vi "FPGA VI_16 Channels.vi"() -> ()   [LabVIEW 2015]
uses:
  Types/Injector.Timing.ctl
  Types/Injection.Core.Settings.ctl
  Types/Injection.Global.Settings.ctl
  <vilib>/Platform/TimedLoop/XDataNode/timing_clust.ctl
  <vilib>/Platform/TimedLoop/XDataNode/nitl_modes.ctl
  <vilib>/Platform/TimedLoop/XDataNode/wakeup.ctl
  Types/Injection.Core.Internal.Settings.ctl
  <vilib>/rvi/Emulation/niFpgaGetClockAttributes.vi
  <vilib>/rvi/Emulation/niFpgaSctlEmulationGetInTimedLoop.vi
  <vilib>/rvi/Emulation/niFpgaEmulationReportErrorSimple.vi
  <vilib>/rvi/eio/common/nirviEmuTemplateMethod_errors.vi
  <vilib>/rvi/Emulation/niFpgaCriticalErrorInLSC.vi
  <vilib>/rvi/DataTransferAndStorage/Container/Common/niFpgaContainerExecOnDevCompGetState.vi
  <vilib>/rvi/Emulation/niFpgaEmulationIsFPGAContextNoSignature.vi
  <vilib>/rvi/errors/niFpgaSetErrorForExecOnDevCompSimple.vi
  <vilib>/rvi/eio/common/nirviEmuReportErrorAndStop.vi
  <vilib>/rvi/DataTransferAndStorage/Container/Common/niFpgaContainerGetUniqueNameForEmu.vi
  <vilib>/rvi/FIFO/Fifo_Resource/nirvififoEmulationSetSize.vi
  <vilib>/rvi/FIFO/Fifo_Resource/nirviFifoEmulationQueueMgr.vi
  <instcachedir>/0/nirviFifoEmulationQueueMgr_E5CAEC123FF24DC58D834DCA3CDAA9B5.lvgen/nirviFifoEmulationQueueMgr_E5CAEC123FF24DC58D834DCA3CDAA9B5_010.vi
  <vilib>/rvi/FIFO/Fifo_Resource/nirvififoEmulationDetermineInputValidOut.vi
  <vilib>/rvi/FIFO/Fifo_Resource/nirvififoEmulationCreateLock.vi
  <vilib>/rvi/Emulation/niFpgaProcessEmulError.vi
  <vilib>/rvi/FIFO/Fifo_Resource/nirvififoEmulationObtainLock.vi
  <vilib>/rvi/FIFO/Fifo_Resource/nirvififoEmulationReleaseLock.vi
  <vilib>/rvi/occurrence/nirviWaitOnOccurrenceBase.vi
  <vilib>/rvi/errors/nirviReportUnexpectedCaseInternalError.vi
  <vilib>/rvi/errors/nirviReportUnexpectedCaseInternalError (U32).vi
  <vilib>/Utility/error.llb/Clear Errors.vi
  <vilib>/rvi/interface/RandomDataEmulation/niFpgaRandomDataHandleErrors.vi
  <instcachedir>/0/nirviFifoEmulationQueueMgr_E5CAEC123FF24DC58D834DCA3CDAA9B5.lvgen/nirviFifoEmulationQueueMgr_E5CAEC123FF24DC58D834DCA3CDAA9B5_008.vi
  <vilib>/eio/EIONode/EIONode.xnode
  <vilib>/Platform/TimedLoop/XDataNode/XDataNode.xnode
  <vilib>/rvi/DataTransferAndStorage/Container/XNode/niFpgaContainer.xnode
  <vilib>/rvi/FIFO/Fifo_Resource/niFpgaFifoEmulationRefIn.vi
  <vilib>/rvi/interface/RandomDataEmulation/nirviRandomDataFpgaReadWriteTemplate.vi
  <vilib>/Platform/TimedLoop/XDataNode/XDNodeRunTimeDep.lvlib
panel:
  in  "Settings.Index12.Injector12":T1
  in  "Settings.Index13.Injector13":T1
  in  "Settings.Index14.Injector14":T1
  in  "Settings.Index15.Injector15":T1
  in  "Settings.Index6.Injector6":T1
  in  "Settings.Index7.Injector7":T1
  in  "Settings.Index8.Injector8":T1
  in  "Settings.Index9.Injector9":T1
  in  "Settings.Index10.Injector10":T1
  in  "Settings.Index11.Injector11":T1
  out "Intermediate FIFO Write Timeout":bool
  in  "Settings.Global":T2={"Enable?"=FALSE, "Initial Voltage Threshold"=12.0, "Event Dwell Limit"=2000, "Voltage Gain"=1.0, "Current Gain"=1.0}
  in  "Settings.Index0.Injector0":T1
  in  "Settings.Index1.Injector1":T1
  in  "Settings.Index2.Injector2":T1
  in  "Settings.Index3.Injector3":T1
  in  "Settings.Index4.Injector4":T1
  in  "Settings.Index5.Injector5":T1
  in  "Settings.Timing":T3={"Injector Sample Period (Ticks)"=125}
  out "Acqusition Loop Ticks":u32
  in  "Settings.DMA":cluster{"# of Injectors":u8}={"# of Injectors"=16}
  out "Host DMA Out?":bool
  out "Intermediate Time Out?":bool
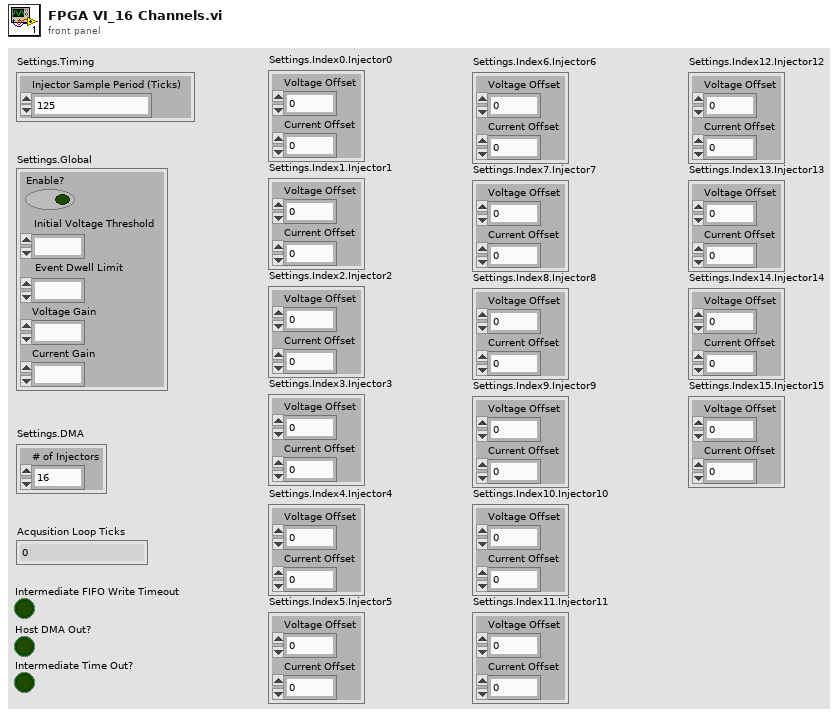
[diagram p1: front panel]
types:
  T1 = typedef "Injection.Core.Settings.ctl" = cluster{"Voltage Offset":fxp<+/-,32,8>, "Current Offset":fxp<+/-,32,8>}
  T2 = typedef "Injection.Global.Settings.ctl" = cluster{"Enable?":bool, "Initial Voltage Threshold":fxp<+/-,32,8>, "Event Dwell Limit":u16, "Voltage Gain":fxp<+/-,32,8>, "Current Gain":fxp<+/-,32,8>}
  T3 = typedef "Injector.Timing.ctl" = cluster{"Injector Sample Period (Ticks)":u32}
  T4 = cluster{"Data.Samples":u32, "Injection.Period":u32, "Injector.Index":u8, "Iteration":u32}
  T5 = enum8{"Wait on Transfer", "Transfer Injector Index", "Transfer # of Samples", "Transfer Injection Period", "Transfer Data Samples"}
  T6 = typedef "XDNodeRunTimeDep.lvlib/timing_clust.ctl" = cluster{"Expected End [f-1]":u64, "Actual End [f-1]":u64, "Finished Late? [f-1]":bool, "Expected End [i-1]":u64, "Actual End [i-1]":u64, "Finished Late? [i-1]":bool, "Expected Start [i]":u64, "Actual Start [i]":u64, "Expected Start [f]":u64, "Actual Start [f]":u64, "Source Name":string, "Structure Name":string, "Period":i64, "Deadline":i64, "Offset":i64, "Start":i64, "Priority":i32, "Timeout":i32, "Mode":T7, "Wakeup Reason":T8, "Error":errorcluster, "Source Type":string, "Secondary Source Type":string, "Global End Time":u64, "Global Start Time":u64, "Frame Duration":u64, "Iteration Duration":u64, "Assigned CPU":i32, "I/O Scan Engine Mode":u32}
  T7 = typedef "XDNodeRunTimeDep.lvlib/nitl_modes.ctl" = enum32{"No Change", "Process missed periods, maintain original phase", "Discard missed periods, maintain original phase", "Process missed periods, ignore original phase", "Discard missed periods, ignore original phase"}
  T8 = typedef "XDNodeRunTimeDep.lvlib/wakeup.ctl" = enum32{"Normal", "Aborted", "Asynchronous wakeup", "Timing source error", "Timed loop error", "Timeout"}
  T9 = typedef "Injection.Core.Internal.Settings.ctl" = cluster{"Data FIFO":refnum<k21>, "Trigger FIFO":refnum<k21>}
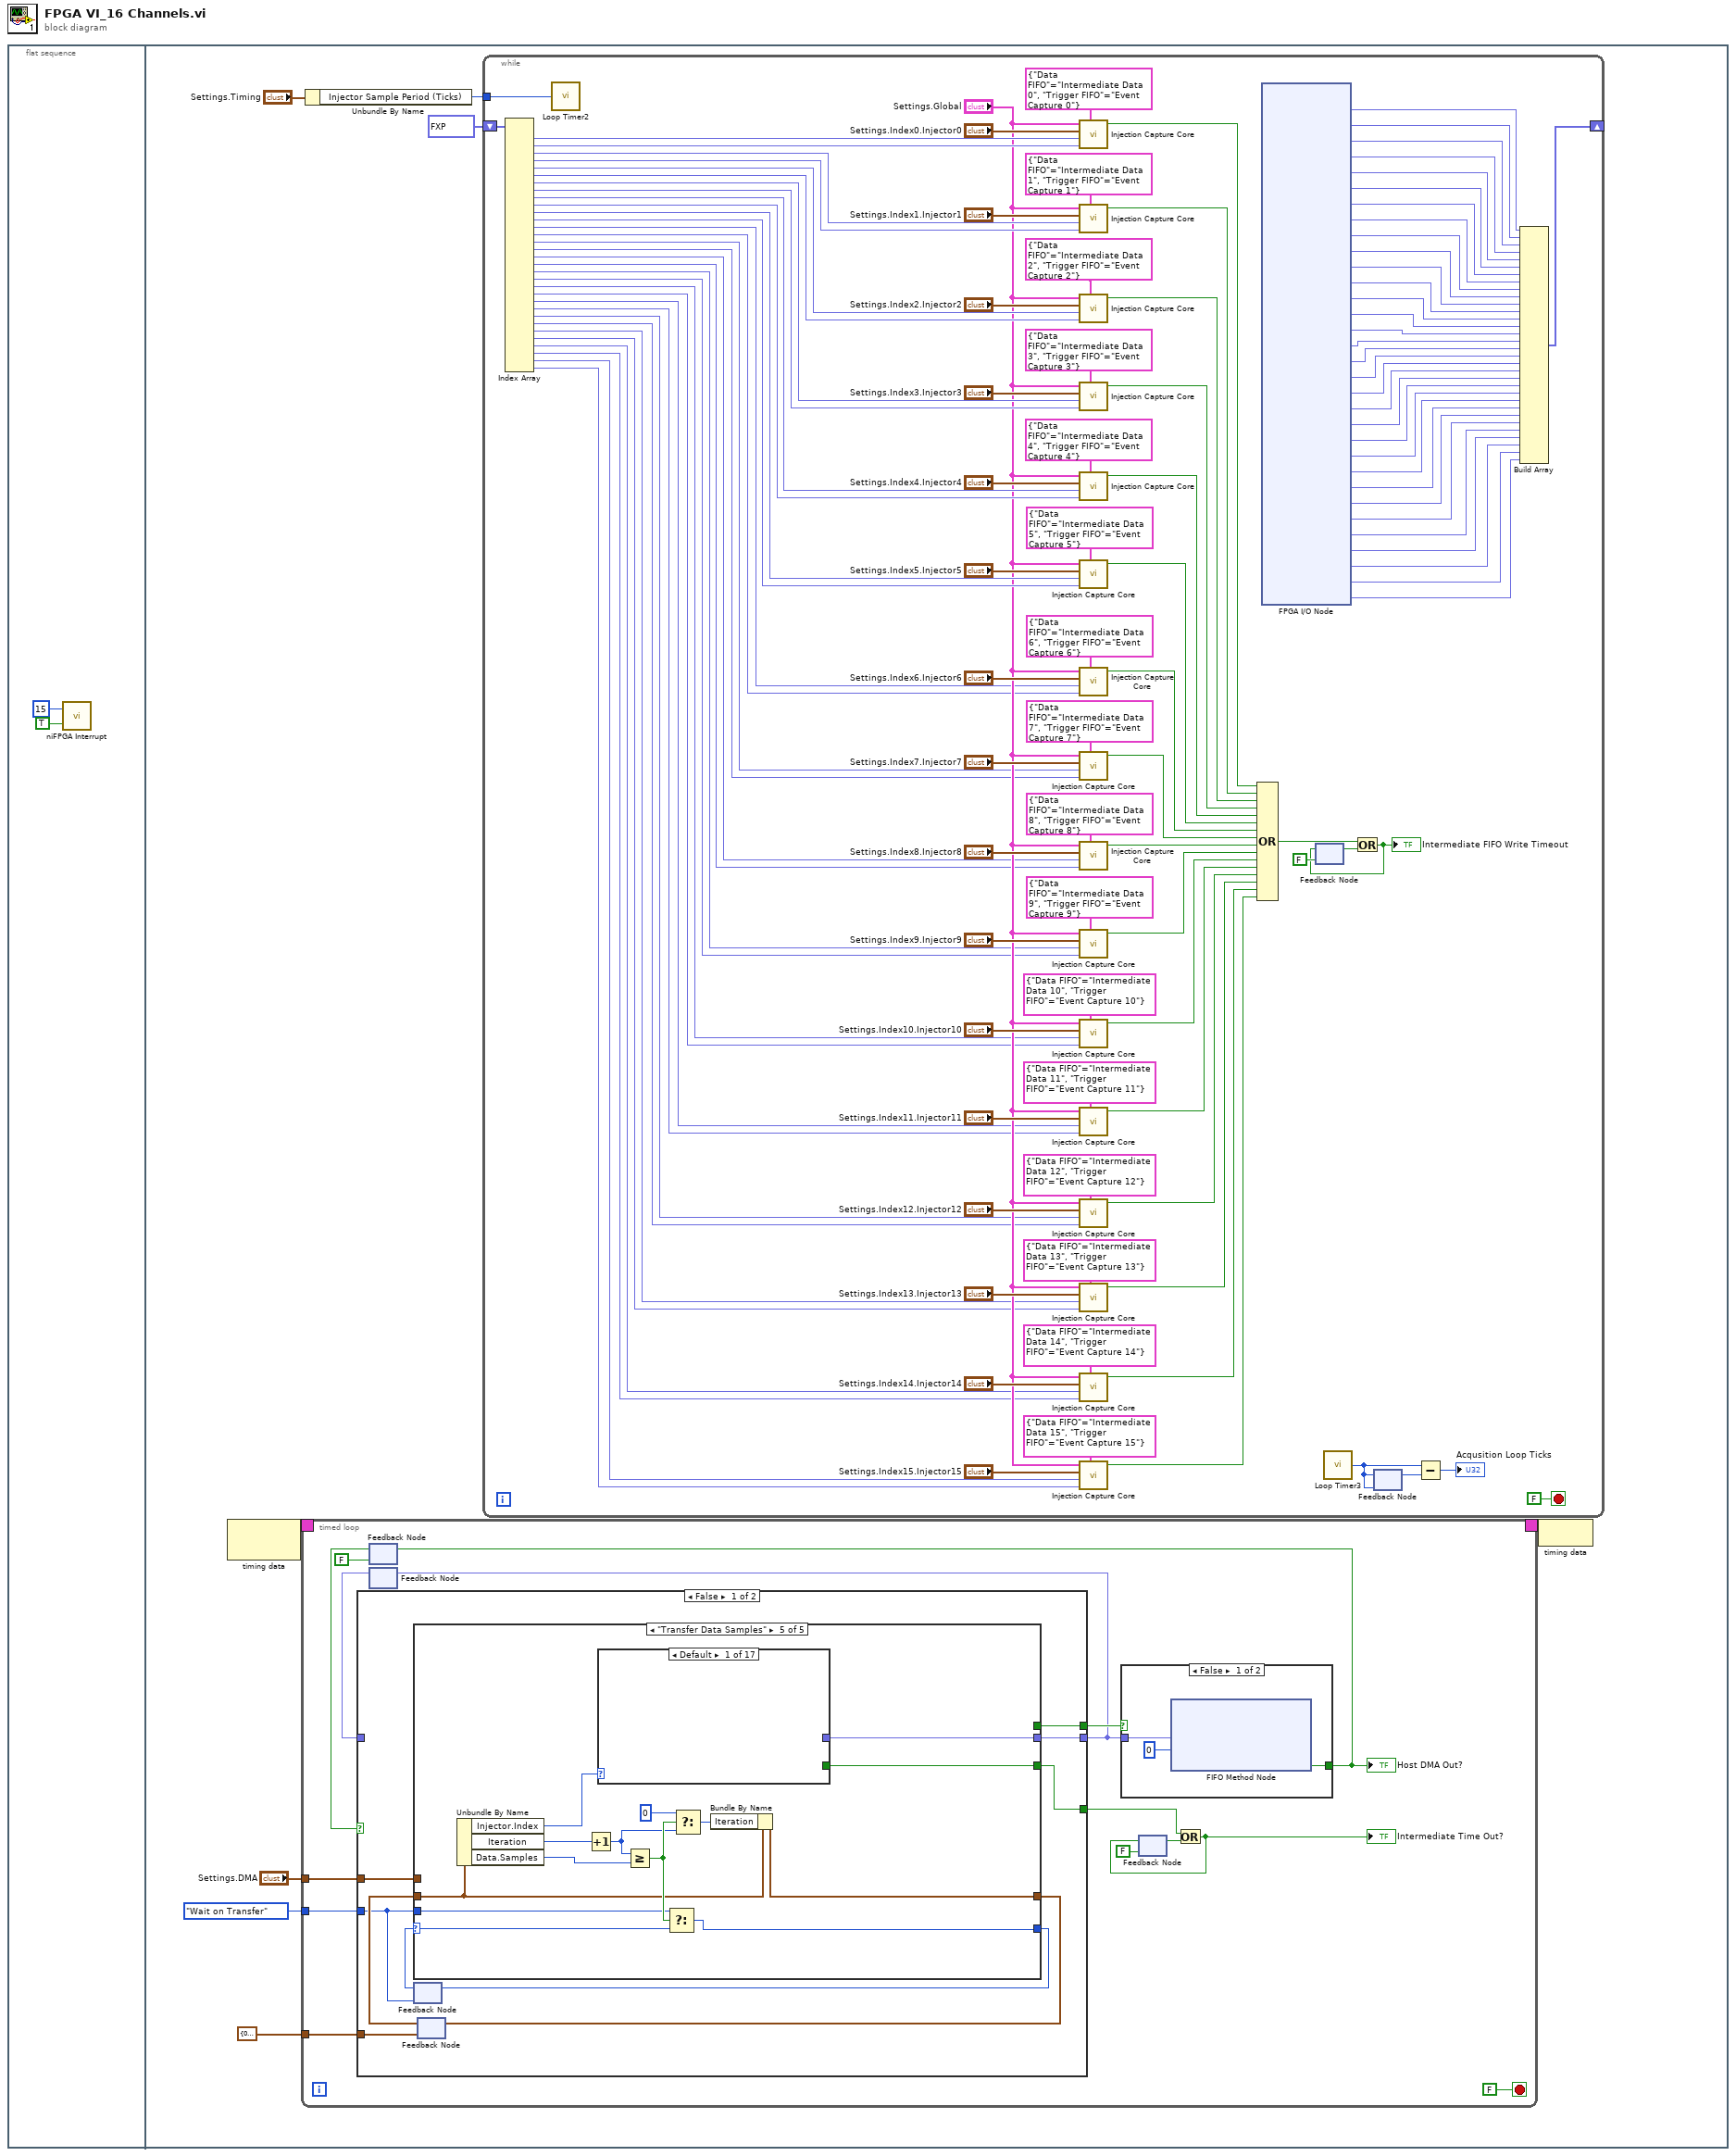
[diagram p0: block diagram]
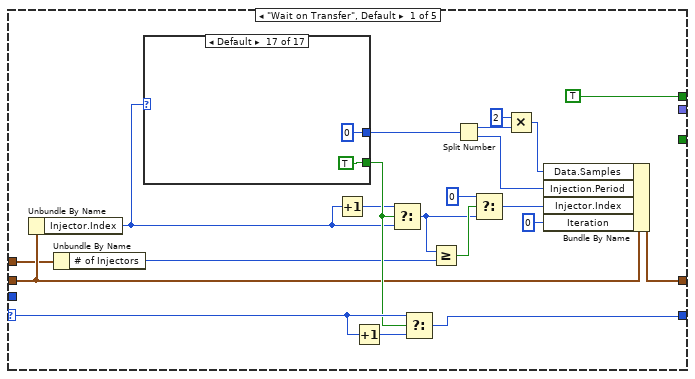
[diagram p2: hidden frame]
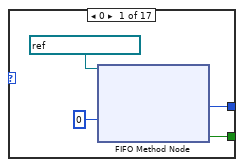
[diagram p3: hidden frame]
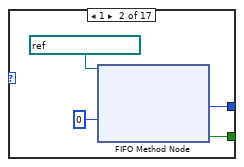
[diagram p4: hidden frame]
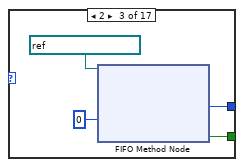
[diagram p5: hidden frame]
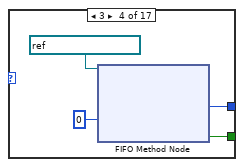
[diagram p6: hidden frame]
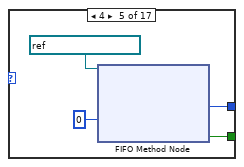
[diagram p7: hidden frame]
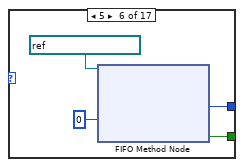
[diagram p8: hidden frame]
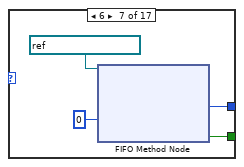
[diagram p9: hidden frame]
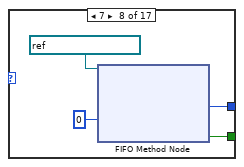
[diagram p10: hidden frame]
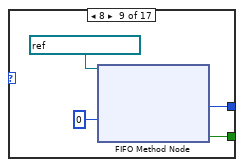
[diagram p11: hidden frame]
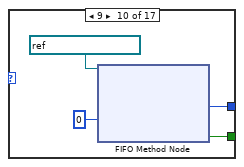
[diagram p12: hidden frame]
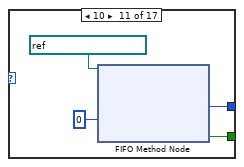
[diagram p13: hidden frame]
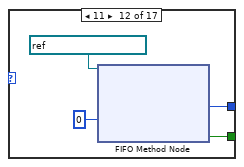
[diagram p14: hidden frame]
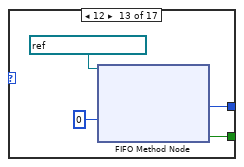
[diagram p15: hidden frame]
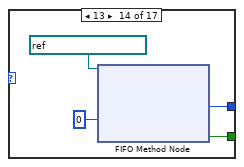
[diagram p16: hidden frame]
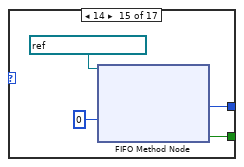
[diagram p17: hidden frame]
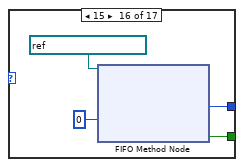
[diagram p18: hidden frame]
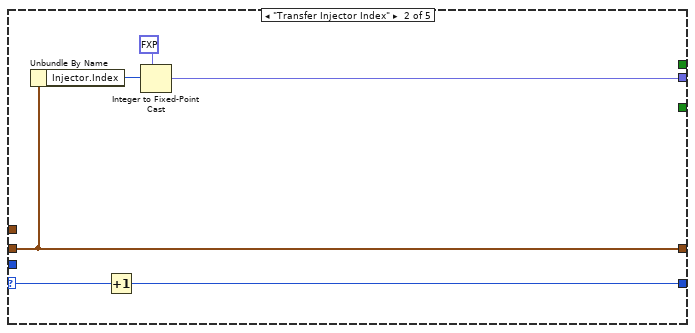
[diagram p19: hidden frame]
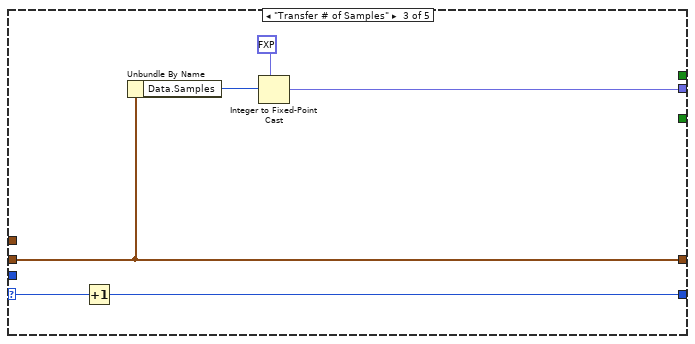
[diagram p20: hidden frame]
diagram:
  n1 = flat-sequence {
    frame #0 {
      n2 = call <vilib>:"niFPGA Interrupt.vi"("Wait Until Cleared (F)"=TRUE, "IRQ Number (0)"=u8 15) -> ()  [unwired: 1 in]
    }
    frame #1 {
      n3 = node-c288() -> (w10:T6)  [unwired: 1 in]
      n4 = timed-loop {
        timing: w10 -> [_]
        timing-out: [_] -> w9
        tunnel: "Settings.DMA" -> [w14]
        tunnel: T5."Wait on Transfer" -> [w13]
        tunnel: T4 {"Data.Samples"=0, "Injection.Period"=0, "Injector.Index"=0, "Iteration"=0} ("Local.Data") -> [w12]
        stop <- FALSE stop-if-true
        n5 = feedback #1(FALSE ("Timed Out?")) -> (w22:bool)
        n6 = feedback #2() -> (w19:fxp<+/-,32,8>)  [unwired: 1 in]
        n7 = case shown="False" w22 {
          tunnel: [w34 w219] -> w20
          tunnel: [w33 w218] -> w24
          tunnel: w13 -> [w26 _]
          tunnel: [w31 w218] -> w15
          tunnel: w14 -> [w30 _]
          tunnel: w12 -> [w27 _]
          tunnel: w19 -> [_ w219]
          frame False {
            n8 = feedback #3(w26) -> (w25:T5)
            n9 = feedback #4(w27) -> (w28:T4)
            n10 = case shown="\"Transfer Data Samples\"" w25 {
              selector: w25 -> [w54 w127 w131 w138 w147]
              tunnel: w28 -> [w45 w124 w129 w135 w145]
              tunnel: [w53 w124 w129 w135 w144] -> w29
              tunnel: [w52 w126 w130 w134 w146] -> w32
              tunnel: [_ w123 w128 w137 w143] -> w34
              tunnel: [TRUE _ _ _ _] -> w33
              tunnel: w26 -> [_ _ _ _ w140]
              tunnel: [_ _ _ _ w142] -> w31
              tunnel: w30 -> [w42 _ _ _ _]
              frame "Wait on Transfer", Default {
                n11 = Unbundle By Name(w45) -> ("Injector.Index"=w44:u8)
                n12 = Unbundle By Name(w42) -> ("# of Injectors"=w41:u8)
                n13 = case shown="Default" w44 {
                  tunnel: [w58 w62 w66 w70 w74 w78 w82 w86 w90 w94 w98 w102 w106 w110 w114 w118 u64 0 ("Element")] -> w40
                  tunnel: [w57 w61 w65 w69 w73 w77 w81 w85 w89 w93 w97 w101 w105 w109 w113 w117 TRUE ("Timed Out?")] -> w50
                  frame 0 {
                    n14 = xnode ("FIFO Method Node")("Timeout"=0, "FIFO In"=refnum<k21> "Event Capture 0") -> ("Element"=w58:u64, "Timed Out?"=w57:bool)  [unwired: 1 out]
                  }
                  frame 1 {
                    n15 = xnode ("FIFO Method Node")("Timeout"=0, "FIFO In"=refnum<k21> "Event Capture 1") -> ("Element"=w62:u64, "Timed Out?"=w61:bool)  [unwired: 1 out]
                  }
                  frame 2 {
                    n16 = xnode ("FIFO Method Node")("Timeout"=0, "FIFO In"=refnum<k21> "Event Capture 2") -> ("Element"=w66:u64, "Timed Out?"=w65:bool)  [unwired: 1 out]
                  }
                  frame 3 {
                    n17 = xnode ("FIFO Method Node")("Timeout"=0, "FIFO In"=refnum<k21> "Event Capture 3") -> ("Element"=w70:u64, "Timed Out?"=w69:bool)  [unwired: 1 out]
                  }
                  frame 4 {
                    n18 = xnode ("FIFO Method Node")("Timeout"=0, "FIFO In"=refnum<k21> "Event Capture 4") -> ("Element"=w74:u64, "Timed Out?"=w73:bool)  [unwired: 1 out]
                  }
                  frame 5 {
                    n19 = xnode ("FIFO Method Node")("Timeout"=0, "FIFO In"=refnum<k21> "Event Capture 5") -> ("Element"=w78:u64, "Timed Out?"=w77:bool)  [unwired: 1 out]
                  }
                  frame 6 {
                    n20 = xnode ("FIFO Method Node")("Timeout"=0, "FIFO In"=refnum<k21> "Event Capture 6") -> ("Element"=w82:u64, "Timed Out?"=w81:bool)  [unwired: 1 out]
                  }
                  frame 7 {
                    n21 = xnode ("FIFO Method Node")("Timeout"=0, "FIFO In"=refnum<k21> "Event Capture 7") -> ("Element"=w86:u64, "Timed Out?"=w85:bool)  [unwired: 1 out]
                  }
                  frame 8 {
                    n22 = xnode ("FIFO Method Node")("Timeout"=0, "FIFO In"=refnum<k21> "Event Capture 8") -> ("Element"=w90:u64, "Timed Out?"=w89:bool)  [unwired: 1 out]
                  }
                  frame 9 {
                    n23 = xnode ("FIFO Method Node")("Timeout"=0, "FIFO In"=refnum<k21> "Event Capture 9") -> ("Element"=w94:u64, "Timed Out?"=w93:bool)  [unwired: 1 out]
                  }
                  frame 10 {
                    n24 = xnode ("FIFO Method Node")("Timeout"=0, "FIFO In"=refnum<k21> "Event Capture 10") -> ("Element"=w98:u64, "Timed Out?"=w97:bool)  [unwired: 1 out]
                  }
                  frame 11 {
                    n25 = xnode ("FIFO Method Node")("Timeout"=0, "FIFO In"=refnum<k21> "Event Capture 11") -> ("Element"=w102:u64, "Timed Out?"=w101:bool)  [unwired: 1 out]
                  }
                  frame 12 {
                    n26 = xnode ("FIFO Method Node")("Timeout"=0, "FIFO In"=refnum<k21> "Event Capture 12") -> ("Element"=w106:u64, "Timed Out?"=w105:bool)  [unwired: 1 out]
                  }
                  frame 13 {
                    n27 = xnode ("FIFO Method Node")("Timeout"=0, "FIFO In"=refnum<k21> "Event Capture 13") -> ("Element"=w110:u64, "Timed Out?"=w109:bool)  [unwired: 1 out]
                  }
                  frame 14 {
                    n28 = xnode ("FIFO Method Node")("Timeout"=0, "FIFO In"=refnum<k21> "Event Capture 14") -> ("Element"=w114:u64, "Timed Out?"=w113:bool)  [unwired: 1 out]
                  }
                  frame 15 {
                    n29 = xnode ("FIFO Method Node")("Timeout"=0, "FIFO In"=refnum<k21> "Event Capture 15") -> ("Element"=w118:u64, "Timed Out?"=w117:bool)  [unwired: 1 out]
                  }
                  frame Default {
                  }
                }
                n30 = Increment(x=w44) -> (x+1=w49:u8)
                n31 = Increment(x=w54) -> (x+1=w55:T5)
                n32 = Select(t=w49, s=w50, f=w44) -> (s? t:f=w47:u8)
                n33 = Select(t=w54, s=w50, f=w55) -> (s? t:f=w52:T5)
                n34 = Greater Or Equal?(x=w47, y=w41) -> (x >= y?=w48:bool)
                n35 = Split Number(x=w40) -> (hi(x)=w39:u32, lo(x)=w38:u32)
                n36 = Select(t=u8 0, s=w48, f=w47) -> (s? t:f=w43:u8)
                n37 = Multiply(x=u32 2, y=w39) -> (x*y=w36:u32)
                n38 = Bundle By Name(cluster=w45, "Data.Samples"=w36, "Injection.Period"=w38, "Injector.Index"=w43, "Iteration"=u32 0) -> (w53:T4)
              }
              frame "Transfer Injector Index" {
                n39 = Unbundle By Name(w124) -> ("Injector.Index"=w125:u8)
                n40 = Increment(x=w127) -> (x+1=w126:T5)
                n41 = Integer to Fixed-Point Cast(fixed-point type=fxp<+/-,32,8> 0.0, integer=w125) -> (fixed-point=w123:fxp<+/-,32,8>)
              }
              frame "Transfer # of Samples" {
                n42 = Increment(x=w131) -> (x+1=w130:T5)
                n43 = Unbundle By Name(w129) -> ("Data.Samples"=w132:u32)
                n44 = Integer to Fixed-Point Cast(fixed-point type=fxp<+/-,32,8> 0.0, integer=w132) -> (fixed-point=w128:fxp<+/-,32,8>)
              }
              frame "Transfer Injection Period" {
                n45 = Unbundle By Name(w135) -> ("Injection.Period"=w136:u32)
                n46 = Increment(x=w138) -> (x+1=w134:T5)
                n47 = Integer to Fixed-Point Cast(fixed-point type=fxp<+/-,32,8> 0.0, integer=w136) -> (fixed-point=w137:fxp<+/-,32,8>)
              }
              frame "Transfer Data Samples" {
                n48 = Unbundle By Name(w145) -> ("Injector.Index"=w153:u8, "Iteration"=w148:u32, "Data.Samples"=w141:u32)
                n49 = Increment(x=w148) -> (x+1=w150:u32)
                n50 = case shown="Default" w153 {
                  tunnel: [_ w156 w160 w164 w168 w172 w176 w180 w184 w188 w192 w196 w200 w204 w208 w212 w216] -> w143
                  tunnel: [_ w155 w159 w163 w167 w171 w175 w179 w183 w187 w191 w195 w199 w203 w207 w211 w215] -> w142
                  frame Default {
                  }
                  frame 0 {
                    n51 = xnode ("FIFO Method Node")("Timeout"=0, "FIFO In"=refnum<k21> "Intermediate Data 0" ("Voltage FIFO")) -> ("Element"=w156:fxp<+/-,32,8>, "Timed Out?"=w155:bool)  [unwired: 1 out]
                  }
                  frame 1 {
                    n52 = xnode ("FIFO Method Node")("Timeout"=0, "FIFO In"=refnum<k21> "Intermediate Data 1" ("Voltage FIFO")) -> ("Element"=w160:fxp<+/-,32,8>, "Timed Out?"=w159:bool)  [unwired: 1 out]
                  }
                  frame 2 {
                    n53 = xnode ("FIFO Method Node")("Timeout"=0, "FIFO In"=refnum<k21> "Intermediate Data 2" ("Voltage FIFO")) -> ("Element"=w164:fxp<+/-,32,8>, "Timed Out?"=w163:bool)  [unwired: 1 out]
                  }
                  frame 3 {
                    n54 = xnode ("FIFO Method Node")("Timeout"=0, "FIFO In"=refnum<k21> "Intermediate Data 3" ("Voltage FIFO")) -> ("Element"=w168:fxp<+/-,32,8>, "Timed Out?"=w167:bool)  [unwired: 1 out]
                  }
                  frame 4 {
                    n55 = xnode ("FIFO Method Node")("Timeout"=0, "FIFO In"=refnum<k21> "Intermediate Data 4" ("Voltage FIFO")) -> ("Element"=w172:fxp<+/-,32,8>, "Timed Out?"=w171:bool)  [unwired: 1 out]
                  }
                  frame 5 {
                    n56 = xnode ("FIFO Method Node")("Timeout"=0, "FIFO In"=refnum<k21> "Intermediate Data 5" ("Voltage FIFO")) -> ("Element"=w176:fxp<+/-,32,8>, "Timed Out?"=w175:bool)  [unwired: 1 out]
                  }
                  frame 6 {
                    n57 = xnode ("FIFO Method Node")("Timeout"=0, "FIFO In"=refnum<k21> "Intermediate Data 6" ("Voltage FIFO")) -> ("Element"=w180:fxp<+/-,32,8>, "Timed Out?"=w179:bool)  [unwired: 1 out]
                  }
                  frame 7 {
                    n58 = xnode ("FIFO Method Node")("Timeout"=0, "FIFO In"=refnum<k21> "Intermediate Data 7" ("Voltage FIFO")) -> ("Element"=w184:fxp<+/-,32,8>, "Timed Out?"=w183:bool)  [unwired: 1 out]
                  }
                  frame 8 {
                    n59 = xnode ("FIFO Method Node")("Timeout"=0, "FIFO In"=refnum<k21> "Intermediate Data 8" ("Voltage FIFO")) -> ("Element"=w188:fxp<+/-,32,8>, "Timed Out?"=w187:bool)  [unwired: 1 out]
                  }
                  frame 9 {
                    n60 = xnode ("FIFO Method Node")("Timeout"=0, "FIFO In"=refnum<k21> "Intermediate Data 9" ("Voltage FIFO")) -> ("Element"=w192:fxp<+/-,32,8>, "Timed Out?"=w191:bool)  [unwired: 1 out]
                  }
                  frame 10 {
                    n61 = xnode ("FIFO Method Node")("Timeout"=0, "FIFO In"=refnum<k21> "Intermediate Data 10" ("Voltage FIFO")) -> ("Element"=w196:fxp<+/-,32,8>, "Timed Out?"=w195:bool)  [unwired: 1 out]
                  }
                  frame 11 {
                    n62 = xnode ("FIFO Method Node")("Timeout"=0, "FIFO In"=refnum<k21> "Intermediate Data 11" ("Voltage FIFO")) -> ("Element"=w200:fxp<+/-,32,8>, "Timed Out?"=w199:bool)  [unwired: 1 out]
                  }
                  frame 12 {
                    n63 = xnode ("FIFO Method Node")("Timeout"=0, "FIFO In"=refnum<k21> "Intermediate Data 12" ("Voltage FIFO")) -> ("Element"=w204:fxp<+/-,32,8>, "Timed Out?"=w203:bool)  [unwired: 1 out]
                  }
                  frame 13 {
                    n64 = xnode ("FIFO Method Node")("Timeout"=0, "FIFO In"=refnum<k21> "Intermediate Data 13" ("Voltage FIFO")) -> ("Element"=w208:fxp<+/-,32,8>, "Timed Out?"=w207:bool)  [unwired: 1 out]
                  }
                  frame 14 {
                    n65 = xnode ("FIFO Method Node")("Timeout"=0, "FIFO In"=refnum<k21> "Intermediate Data 14" ("Voltage FIFO")) -> ("Element"=w212:fxp<+/-,32,8>, "Timed Out?"=w211:bool)  [unwired: 1 out]
                  }
                  frame 15 {
                    n66 = xnode ("FIFO Method Node")("Timeout"=0, "FIFO In"=refnum<k21> "Intermediate Data 15" ("Voltage FIFO")) -> ("Element"=w216:fxp<+/-,32,8>, "Timed Out?"=w215:bool)  [unwired: 1 out]
                  }
                }
                n67 = Greater Or Equal?(x=w150, y=w141) -> (x >= y?=w152:bool)
                n68 = Select(t=w140, s=w152, f=w147) -> (s? t:f=w146:T5)
                n69 = Select(t=u32 0, s=w152, f=w150) -> (s? t:f=w149:u32)
                n70 = Bundle By Name(cluster=w145, "Iteration"=w149) -> (w144:T4)
              }
            }
            n71 = feedback-in #3(w32) -> ()
            n72 = feedback-in #4(w29) -> ()
          }
          frame True {
            w218 = FALSE
          }
        }
        n73 = feedback-in #2(w20) -> ()
        n74 = case shown="False" w24 {
          tunnel: w20 -> [w221 _]
          tunnel: [w220 FALSE ("Timed Out?")] -> w23
          frame False {
            n75 = xnode ("FIFO Method Node")("Element"=w221, "Timeout"=0) -> ("Timed Out?"=w220:bool)  [unwired: 1 in, 1 out]
          }
          frame True {
          }
        }
        "Host DMA Out?" <- w23
        n76 = feedback-in #1(w23) -> ()
        n77 = feedback #5(FALSE ("Timed Out?")) -> (w17:bool)
        n78 = Or(x=w15, y=w17) -> (x .or. y?=w16:bool)
        "Intermediate Time Out?" <- w16
        n79 = feedback-in #5(w16) -> ()
      }
      n80 = Unbundle By Name("Settings.Timing") -> ("Injector Sample Period (Ticks)"=w3:u32)
      n81 = while {
        shift-right: [w311] -> _
        shift-left: fxp<+/-,24,5>[] [0.0, 0.0, 0.0, 0.0, 0.0, 0.0, 0.0, 0.0, 0.0, 0.0, 0.0, 0.0, 0.0, 0.0, 0.0, 0.0, 0.0, 0.0, 0.0, 0.0, 0.0, 0.0, 0.0, 0.0, 0.0, 0.0, 0.0, 0.0, 0.0, 0.0, 0.0, 0.0] -> [w332]
        tunnel: w3 -> [w317]
        stop <- FALSE stop-if-true
        n82 = Index Array(array=w332) -> (element #1=w343:fxp<+/-,24,5>, element #2=w344:fxp<+/-,24,5>, element #3=w341:fxp<+/-,24,5>, element #4=w342:fxp<+/-,24,5>, element #5=w339:fxp<+/-,24,5>, element #6=w340:fxp<+/-,24,5>, element #7=w337:fxp<+/-,24,5>, element #8=w338:fxp<+/-,24,5>, element #9=w335:fxp<+/-,24,5>, element #10=w336:fxp<+/-,24,5>, element #11=w333:fxp<+/-,24,5>, element #12=w334:fxp<+/-,24,5>, element #13=w247:fxp<+/-,24,5>, element #14=w246:fxp<+/-,24,5>, element #15=w245:fxp<+/-,24,5>, element #16=w244:fxp<+/-,24,5>, element #17=w243:fxp<+/-,24,5>, element #18=w242:fxp<+/-,24,5>, element #19=w241:fxp<+/-,24,5>, element #20=w240:fxp<+/-,24,5>, element #21=w239:fxp<+/-,24,5>, element #22=w238:fxp<+/-,24,5>, element #23=w237:fxp<+/-,24,5>, element #24=w236:fxp<+/-,24,5>, element #25=w235:fxp<+/-,24,5>, element #26=w234:fxp<+/-,24,5>, element #27=w233:fxp<+/-,24,5>, element #28=w232:fxp<+/-,24,5>, element #29=w231:fxp<+/-,24,5>, element #30=w230:fxp<+/-,24,5>, element #31=w229:fxp<+/-,24,5>, element #32=w228:fxp<+/-,24,5>)  [unwired: 32 in]
        n83 = call "Loop Timer2"("Count(Ticks)"=w317) -> ()  [unwired: 1 out]
        n84 = call "Injection Capture Core.vi"("FIFOs"=T9 {"Data FIFO"="Intermediate Data 0", "Trigger FIFO"="Event Capture 0"} ("InjectorCore.Settings"), "Current (PreScaled)"=w344, "Voltage (PreScaled)"=w343, "Settings.Index<#>.<UserName>"="Settings.Index0.Injector0", "Settings.Global"="Settings.Global") -> ("Intermediate FIFO Timeout?"=w351:bool)  [unwired: 4 in, 2 out]
        n85 = call "Injection Capture Core.vi"("FIFOs"=T9 {"Data FIFO"="Intermediate Data 1", "Trigger FIFO"="Event Capture 1"} ("InjectorCore.Settings"), "Current (PreScaled)"=w342, "Voltage (PreScaled)"=w341, "Settings.Index<#>.<UserName>"="Settings.Index1.Injector1", "Settings.Global"="Settings.Global") -> ("Intermediate FIFO Timeout?"=w350:bool)  [unwired: 4 in, 2 out]
        n86 = call "Injection Capture Core.vi"("FIFOs"=T9 {"Data FIFO"="Intermediate Data 2", "Trigger FIFO"="Event Capture 2"} ("InjectorCore.Settings"), "Current (PreScaled)"=w340, "Voltage (PreScaled)"=w339, "Settings.Index<#>.<UserName>"="Settings.Index2.Injector2", "Settings.Global"="Settings.Global") -> ("Intermediate FIFO Timeout?"=w349:bool)  [unwired: 4 in, 2 out]
        n87 = call "Injection Capture Core.vi"("FIFOs"=T9 {"Data FIFO"="Intermediate Data 3", "Trigger FIFO"="Event Capture 3"} ("InjectorCore.Settings"), "Current (PreScaled)"=w338, "Voltage (PreScaled)"=w337, "Settings.Index<#>.<UserName>"="Settings.Index3.Injector3", "Settings.Global"="Settings.Global") -> ("Intermediate FIFO Timeout?"=w348:bool)  [unwired: 4 in, 2 out]
        n88 = call "Injection Capture Core.vi"("FIFOs"=T9 {"Data FIFO"="Intermediate Data 4", "Trigger FIFO"="Event Capture 4"} ("InjectorCore.Settings"), "Current (PreScaled)"=w336, "Voltage (PreScaled)"=w335, "Settings.Index<#>.<UserName>"="Settings.Index4.Injector4", "Settings.Global"="Settings.Global") -> ("Intermediate FIFO Timeout?"=w347:bool)  [unwired: 4 in, 2 out]
        n89 = call "Injection Capture Core.vi"("FIFOs"=T9 {"Data FIFO"="Intermediate Data 5", "Trigger FIFO"="Event Capture 5"} ("InjectorCore.Settings"), "Current (PreScaled)"=w334, "Voltage (PreScaled)"=w333, "Settings.Index<#>.<UserName>"="Settings.Index5.Injector5", "Settings.Global"="Settings.Global") -> ("Intermediate FIFO Timeout?"=w346:bool)  [unwired: 4 in, 2 out]
        n90 = call "Injection Capture Core.vi"("FIFOs"=T9 {"Data FIFO"="Intermediate Data 6", "Trigger FIFO"="Event Capture 6"} ("InjectorCore.Settings"), "Current (PreScaled)"=w246, "Voltage (PreScaled)"=w247, "Settings.Index<#>.<UserName>"="Settings.Index6.Injector6", "Settings.Global"="Settings.Global") -> ("Intermediate FIFO Timeout?"=w257:bool)  [unwired: 4 in, 2 out]
        n91 = call "Injection Capture Core.vi"("FIFOs"=T9 {"Data FIFO"="Intermediate Data 7", "Trigger FIFO"="Event Capture 7"} ("InjectorCore.Settings"), "Current (PreScaled)"=w244, "Voltage (PreScaled)"=w245, "Settings.Index<#>.<UserName>"="Settings.Index7.Injector7", "Settings.Global"="Settings.Global") -> ("Intermediate FIFO Timeout?"=w256:bool)  [unwired: 4 in, 2 out]
        n92 = call "Injection Capture Core.vi"("FIFOs"=T9 {"Data FIFO"="Intermediate Data 8", "Trigger FIFO"="Event Capture 8"} ("InjectorCore.Settings"), "Current (PreScaled)"=w242, "Voltage (PreScaled)"=w243, "Settings.Index<#>.<UserName>"="Settings.Index8.Injector8", "Settings.Global"="Settings.Global") -> ("Intermediate FIFO Timeout?"=w255:bool)  [unwired: 4 in, 2 out]
        n93 = call "Injection Capture Core.vi"("FIFOs"=T9 {"Data FIFO"="Intermediate Data 9", "Trigger FIFO"="Event Capture 9"} ("InjectorCore.Settings"), "Current (PreScaled)"=w240, "Voltage (PreScaled)"=w241, "Settings.Index<#>.<UserName>"="Settings.Index9.Injector9", "Settings.Global"="Settings.Global") -> ("Intermediate FIFO Timeout?"=w254:bool)  [unwired: 4 in, 2 out]
        n94 = call "Injection Capture Core.vi"("FIFOs"=T9 {"Data FIFO"="Intermediate Data 10", "Trigger FIFO"="Event Capture 10"} ("InjectorCore.Settings"), "Current (PreScaled)"=w238, "Voltage (PreScaled)"=w239, "Settings.Index<#>.<UserName>"="Settings.Index10.Injector10", "Settings.Global"="Settings.Global") -> ("Intermediate FIFO Timeout?"=w253:bool)  [unwired: 4 in, 2 out]
        n95 = call "Injection Capture Core.vi"("FIFOs"=T9 {"Data FIFO"="Intermediate Data 11", "Trigger FIFO"="Event Capture 11"} ("InjectorCore.Settings"), "Current (PreScaled)"=w236, "Voltage (PreScaled)"=w237, "Settings.Index<#>.<UserName>"="Settings.Index11.Injector11", "Settings.Global"="Settings.Global") -> ("Intermediate FIFO Timeout?"=w252:bool)  [unwired: 4 in, 2 out]
        n96 = call "Injection Capture Core.vi"("FIFOs"=T9 {"Data FIFO"="Intermediate Data 12", "Trigger FIFO"="Event Capture 12"} ("InjectorCore.Settings"), "Current (PreScaled)"=w234, "Voltage (PreScaled)"=w235, "Settings.Index<#>.<UserName>"="Settings.Index12.Injector12", "Settings.Global"="Settings.Global") -> ("Intermediate FIFO Timeout?"=w251:bool)  [unwired: 4 in, 2 out]
        n97 = call "Injection Capture Core.vi"("FIFOs"=T9 {"Data FIFO"="Intermediate Data 13", "Trigger FIFO"="Event Capture 13"} ("InjectorCore.Settings"), "Current (PreScaled)"=w232, "Voltage (PreScaled)"=w233, "Settings.Index<#>.<UserName>"="Settings.Index13.Injector13", "Settings.Global"="Settings.Global") -> ("Intermediate FIFO Timeout?"=w250:bool)  [unwired: 4 in, 2 out]
        n98 = call "Injection Capture Core.vi"("FIFOs"=T9 {"Data FIFO"="Intermediate Data 14", "Trigger FIFO"="Event Capture 14"} ("InjectorCore.Settings"), "Current (PreScaled)"=w230, "Voltage (PreScaled)"=w231, "Settings.Index<#>.<UserName>"="Settings.Index14.Injector14", "Settings.Global"="Settings.Global") -> ("Intermediate FIFO Timeout?"=w249:bool)  [unwired: 4 in, 2 out]
        n99 = call "Injection Capture Core.vi"("FIFOs"=T9 {"Data FIFO"="Intermediate Data 15", "Trigger FIFO"="Event Capture 15"} ("InjectorCore.Settings"), "Current (PreScaled)"=w228, "Voltage (PreScaled)"=w229, "Settings.Index<#>.<UserName>"="Settings.Index15.Injector15", "Settings.Global"="Settings.Global") -> ("Intermediate FIFO Timeout?"=w248:bool)  [unwired: 4 in, 2 out]
        n100 = Compound Arithmetic op=OR(w351, w350, w349, w348, w347, w346, w257, w256, w255, w254, w253, w252, w251, w250, w249, w248) -> (w322:bool)
        n101 = xnode "FPGA I/O Node"() -> ("Mod1/AI0"=w310:fxp<+/-,24,5>, "Mod1/AI1"=w309:fxp<+/-,24,5>, "Mod1/AI2"=w308:fxp<+/-,24,5>, "Mod1/AI3"=w307:fxp<+/-,24,5>, "Mod2/AI0"=w306:fxp<+/-,24,5>, "Mod2/AI1"=w305:fxp<+/-,24,5>, "Mod2/AI2"=w304:fxp<+/-,24,5>, "Mod2/AI3"=w303:fxp<+/-,24,5>, "Mod3/AI0"=w302:fxp<+/-,24,5>, "Mod3/AI1"=w301:fxp<+/-,24,5>, "Mod3/AI2"=w300:fxp<+/-,24,5>, "Mod3/AI3"=w299:fxp<+/-,24,5>, "Mod4/AI0"=w298:fxp<+/-,24,5>, "Mod4/AI1"=w297:fxp<+/-,24,5>, "Mod4/AI2"=w296:fxp<+/-,24,5>, "Mod4/AI3"=w295:fxp<+/-,24,5>, "Mod5/AI0"=w294:fxp<+/-,24,5>, "Mod5/AI1"=w293:fxp<+/-,24,5>, "Mod5/AI2"=w292:fxp<+/-,24,5>, "Mod5/AI3"=w291:fxp<+/-,24,5>, "Mod6/AI0"=w290:fxp<+/-,24,5>, "Mod6/AI1"=w289:fxp<+/-,24,5>, "Mod6/AI2"=w288:fxp<+/-,24,5>, "Mod6/AI3"=w287:fxp<+/-,24,5>, "Mod7/AI0"=w286:fxp<+/-,24,5>, "Mod7/AI1"=w285:fxp<+/-,24,5>, "Mod7/AI2"=w284:fxp<+/-,24,5>, "Mod7/AI3"=w283:fxp<+/-,24,5>, "Mod8/AI0"=w282:fxp<+/-,24,5>, "Mod8/AI1"=w281:fxp<+/-,24,5>, "Mod8/AI2"=w280:fxp<+/-,24,5>, "Mod8/AI3"=w279:fxp<+/-,24,5>)  [unwired: 32 in, 32 out]
        n102 = feedback #6(FALSE ("Timed Out?")) -> (w323:bool)
        n103 = call "Loop Timer3"() -> ("Tick Count(Ticks)"=w318:u32)  [unwired: 1 in]
        n104 = Or(x=w322, y=w323) -> (x .or. y?=w321:bool)
        "Intermediate FIFO Write Timeout" <- w321
        n105 = feedback-in #6(w321) -> ()
        n106 = feedback-in #7(w318) -> ()
        n107 = feedback #7(w318) -> (w320:u32)
        n108 = Subtract(x=w318, y=w320) -> (x-y=→"Acqusition Loop Ticks":u32)
        n109 = Build Array(w310, w309, w308, w307, w306, w305, w304, w303, w302, w301, w300, w299, w298, w297, w296, w295, w294, w293, w292, w291, w290, w289, w288, w287, w286, w285, w284, w283, w282, w281, w280, w279) -> (w311:fxp<+/-,24,5>[])
      }
      n110 = node-c288(w9) -> ()
    }
  }
